vi "Title-Set.vi"(8 "error in (no error)":errorcluster, 10 "Title":string, 11 "WindowBuilder in":refnum<class "WindowBuilder.lvclass">) -> (0 "error out":errorcluster, 3 "WindowBuilder out":refnum<class "WindowBuilder.lvclass">)   [LabVIEW 2020, in "GLF.lvlib" / "WindowBuilder.lvclass"]
uses:
  WindowBuilder.lvclass
  WindowBuilder.lvclass/WindowBuilder.ctl
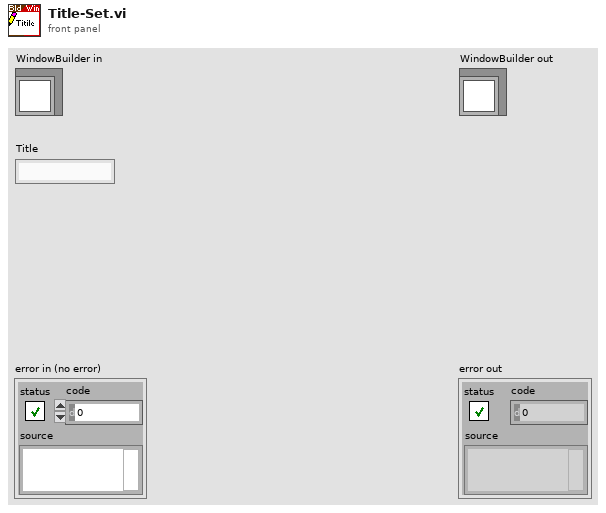
[diagram p1: front panel]
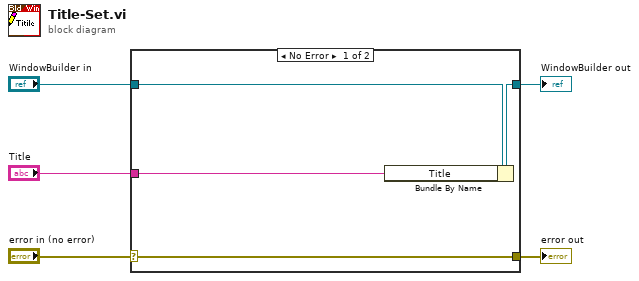
[diagram p0: block diagram]
diagram:
  n1 = case shown="No Error" "error in (no error)" {
    selector: "error in (no error)" -> [w9 w10]
    tunnel: [w9 w10] -> w4
    tunnel: [w7 w11] -> w2
    tunnel: "WindowBuilder in" -> [w8 w11]
    tunnel: "Title" -> [w6 _]
    frame No Error {
      n2 = Bundle By Name(cluster=w8, "Title"=w6) -> (w7:refnum<class "WindowBuilder.lvclass">)
    }
    frame Error {
    }
  }
  "error out" <- w4
  "WindowBuilder out" <- w2
